vi "To File (Path).vi"(5 "access (0:read/write)":enum16{"read/write", "read-only", "write-only"}(ring), 6 "Pretty Print?":bool, 7 "enable LabVIEW extensions? (T)":bool=TRUE, 8 "error in (no error)":errorcluster, 9 "operation (0:open)":T1(ring), 10 "JSON in":refnum<class "JSON Value.lvclass">, 11 "file path":path) -> (0 "error out":errorcluster)   [LabVIEW 2016, in "JSON Value.lvclass"]
doc: "Saves a JSON instance's data to the given file."
uses:
  JSON Value.lvclass
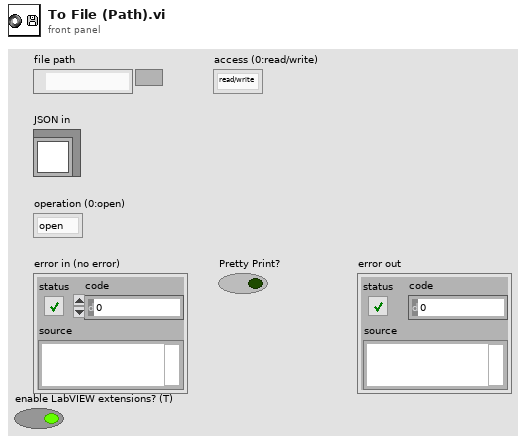
[diagram p1: front panel]
types:
  T1 = enum16{"open", "replace", "create", "open or create", "replace or create", "replace or create with confirmation"}
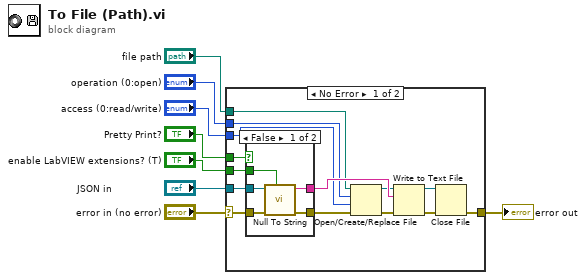
[diagram p0: block diagram]
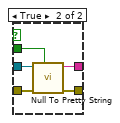
[diagram p2: hidden frame]
diagram:
  n1 = case shown="No Error" "error in (no error)" {
    selector: "error in (no error)" -> [w17 w33]
    tunnel: "JSON in" -> [w22 _]
    tunnel: "file path" -> [w15 _]
    tunnel: [w11 w33] -> w5
    tunnel: "operation (0:open)" -> [w14 _]
    tunnel: "access (0:read/write)" -> [w13 _]
    tunnel: "Pretty Print?" -> [w12 _]
    tunnel: "enable LabVIEW extensions? (T)" -> [w9 _]
    frame No Error {
      n2 = case shown="False" w12 {
        tunnel: w22 -> [w27 w30]
        tunnel: [w26 w29] -> w21
        tunnel: w17 -> [w25 w31]
        tunnel: [w24 w32] -> w10
        tunnel: w9 -> [w23 w28]
        frame False {
          n3 = call "Null To String.vi"("enable LabVIEW extensions? (T)"=w23, "error in (no error)"=w25, "JSON Datatype in"=w27) -> ("error out"=w24:errorcluster, "String"=w26:string)  [unwired: 7 in]
        }
        frame True {
          n4 = call "Null To Pretty String.vi"("enable LabVIEW extensions? (T)"=w28, "error in (no error)"=w31, "JSON Datatype in"=w30) -> ("error out"=w32:errorcluster, "Pretty Print String"=w29:string)  [unwired: 7 in]
        }
      }
      n5 = Open/Create/Replace File(file path (use dialog)=w15, error in=w10, operation (0:open)=w14, access (0:read/write)=w13) -> (refnum out=w18:refnum<file>, error out=w16:errorcluster)  [unwired: 2 in, 1 out]
      n6 = Write to Text File(file (use dialog)=w18, text=w21, error in=w16) -> (refnum out=w19:refnum<file>, error out=w20:errorcluster)  [unwired: 1 in, 1 out]
      n7 = Close File(refnum=w19, error in=w20) -> (error out=w11:errorcluster)  [unwired: 1 out]
    }
    frame Error {
    }
  }
  "error out" <- w5
